vi "Open 2601B.vi"(8 "错误输入（无错误）":errorcluster) -> (0 "错误输出":errorcluster, 3 "退出":bool)   [LabVIEW 2020]
uses:
  VISA 2601B.vi
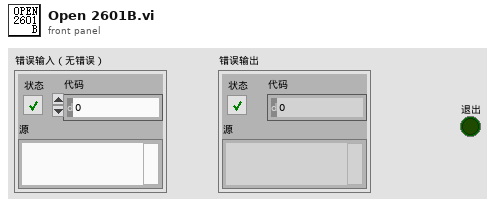
[diagram p1: front panel]
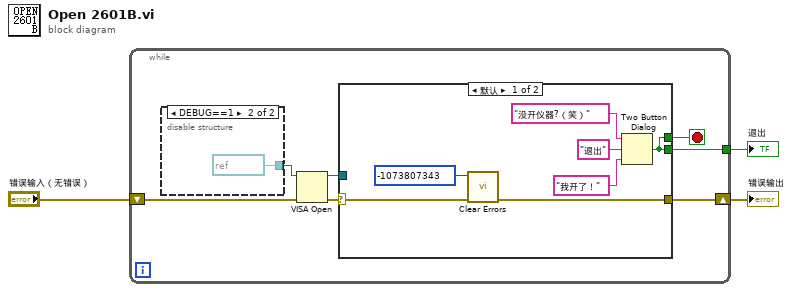
[diagram p0: block diagram]
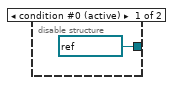
[diagram p2: hidden frame]
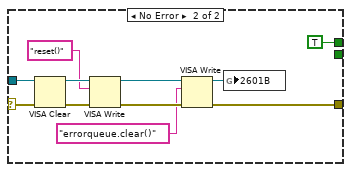
[diagram p3: hidden frame]
diagram:
  n1 = while {
    shift-right: [w10] -> w2
    shift-left: "错误输入（无错误）" -> [w6]
    tunnel: [w8] -> w1
    stop <- w9 stop-if-true
    n2 = disable-structure shown="DEBUG==1" {
      disable-tunnel: [refnum<visa-resource-name> "2601B" ("VISA资源名称") refnum<visa-resource-name> "Test" ("VISA资源名称")] -> w4
      frame condition #0 (active) {
      }
      frame condition #1 {
      }
    }
    n3 = VISA Open(error in (no error)=w6, VISA resource name=w4) -> (VISA resource name=w7:refnum<visa-resource-name>, error out=w5:errorcluster)  [unwired: 3 in]
    n4 = case shown="默认" w5 {
      selector: w5 -> [w18 w20]
      tunnel: [w16 w23] -> w10
      tunnel: [w13 TRUE] -> w9
      tunnel: [w13 _] -> w8
      tunnel: w7 -> [_ w21]
      frame Default {
        n5 = call <vilib>:"Clear Errors.vi"("error in (no error)"=w18, "specific error code to clear (0: all)"=-1073807343) -> ("error out"=w16:errorcluster)  [unwired: 4 in, 1 out]
        n6 = Two Button Dialog(message="没开仪器?（笑）" ("消息"), 1:"我开了！" ("T按钮名称（“确定”）"), 2:"退出" ("F按钮名称（“取消”）")) -> (T button?=w13:bool)
      }
      frame No Error {
        n7 = VISA Clear(VISA resource name=w21, error in (no error)=w20) -> (VISA resource name out=w30:refnum<visa-resource-name>, error out=w29:errorcluster)
        n8 = VISA Write(VISA resource name=w30, write buffer="reset()" ("写入缓冲区"), error in (no error)=w29) -> (VISA resource name out=w26:refnum<visa-resource-name>, error out=w24:errorcluster)  [unwired: 1 out]
        n9 = VISA Write(VISA resource name=w26, write buffer="errorqueue.clear()" ("写入缓冲区"), error in (no error)=w24) -> (VISA resource name out=w25:refnum<visa-resource-name>, error out=w23:errorcluster)  [unwired: 1 out]
        n10 = global write "VISA 2601B.vi" "2601B"(w25) -> ()
      }
    }
  }
  "错误输出" <- w2
  "退出" <- w1
